vi "comm get user data.vi"(8 "error in (no error)":errorcluster, 11 "Comm Handle":u64) -> (0 "error out":errorcluster, 2 "user data":u32, 3 "dup Comm Handle":u64)   [LabVIEW 2009, in "lvserial.lvlib"]
doc: "Receives the user data. The user data is private data value and is unique per serial port. This value is not used by the serial port library for any purpose."
uses:
  lvserial.lvlib
  x64/Release/lvserial.dll
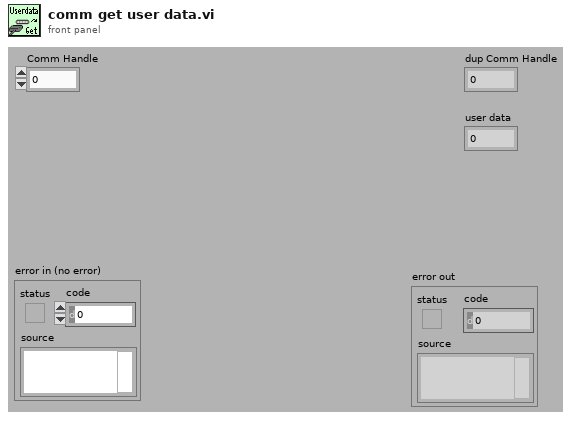
[diagram p1: front panel]
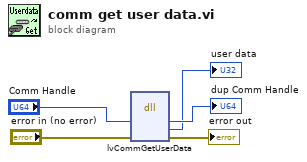
[diagram p0: block diagram]
diagram:
  n1 = dll-call lib="C:/Users/Admin/Desktop/lvserial_source_1-2-13/x64/Release/lvserial.dll" fn="lvCommGetUserData"("hComm"="Comm Handle", "pError"="error in (no error)") -> ("hComm"=→"dup Comm Handle":u64, "pulUserData"=→"user data":u32, "pError"=→"error out":errorcluster)  [unwired: 3 in, 4 out]
